vi "user32_GetMessage.vi"(5 "wMsgFilterMax":u32, 7 "wMsgFilterMin":u32, 8 "错误输入（无错误）":errorcluster, 10 "lpMsg":u32, 11 "hWnd":u32) -> (0 "错误输出":errorcluster, 2 "success?":bool, 3 "dup hWnd":u32)   [LabVIEW 2011]
doc: "函数GetMessage是从调用线程的消息队列里取得一个消息并将其放于指定的结构。此函数可取得与指定窗口联系的消息和由PostThreadMesssge寄送的线程消息。此函数接收一定范围的消息值。GetMessage不接收属于其他线程或应用程序的消息。获取消息成功后，线程将从消息队列中删除该消息。函数会一直等待直到有消息到来才有返回值。"
uses:
  user32.dll
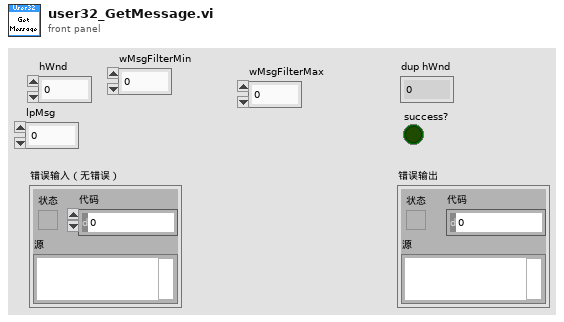
[diagram p1: front panel]
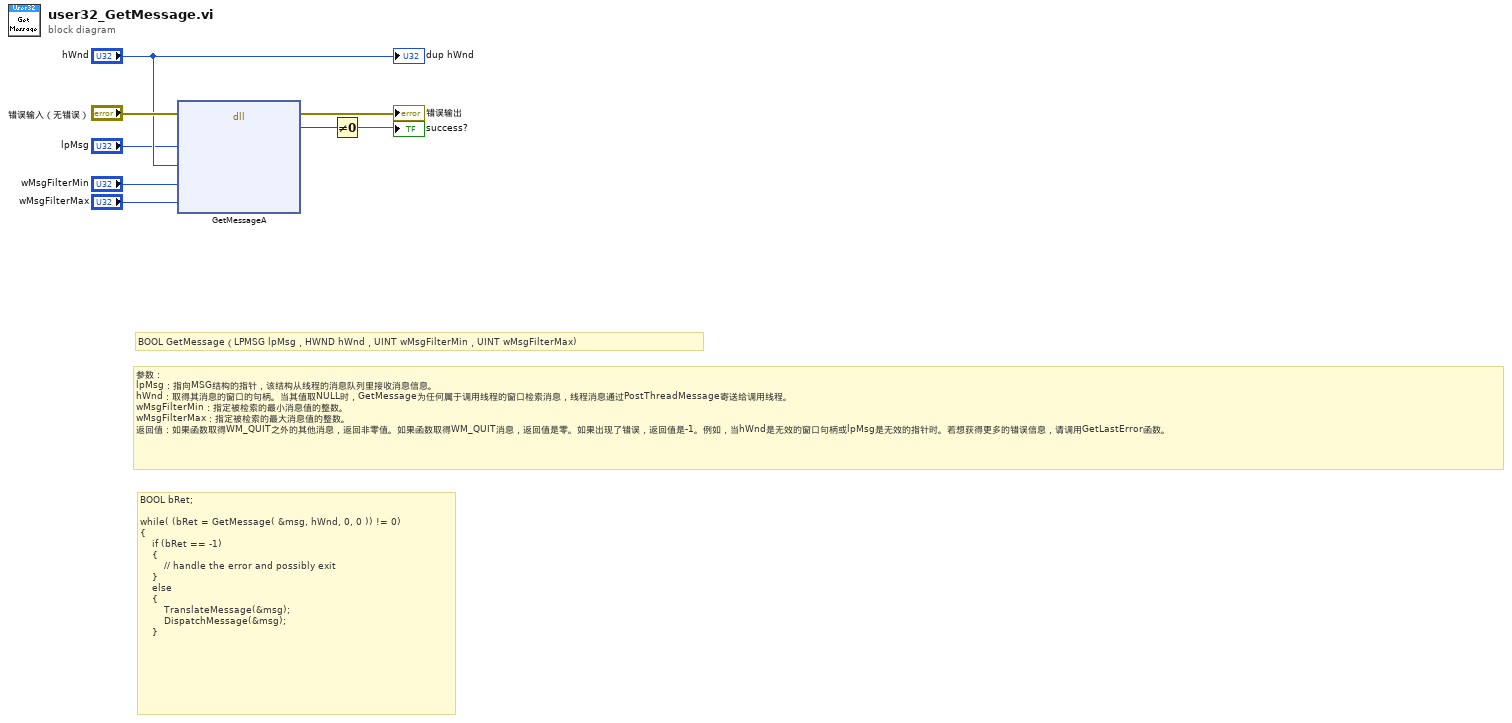
[diagram p0: block diagram]
diagram:
  # "BOOL bRet;\n \nwhile( (bRet = GetMessage( &msg, hWnd, 0, 0 )) != 0)\n{ \n    if (bRet == -1)\n    {\n        // handle the error and possibly exit\n    }\n    else\n    {\n        TranslateMessage(&msg); \n        DispatchMessage(&msg); \n    }"
  # "参数：\nlpMsg：指向MSG结构的指针，该结构从线程的消息队列里接收消息信息。\nhWnd：取得其消息的窗口的句柄。当其值取NULL时，GetMessage为任何属于调用线程的窗口检索消息，线程消息通过PostThreadMessage寄送给调用线程。\nwMsgFilterMin：指定被检索的最小消息值的整数。\nwMsgFilterMax：指定被检索的最大消息值的整数。\n返回值：如果函数取得WM_QUIT之外的其他消息，返回非零值。如果函数取得WM_QUIT消息，返回值是零。如果出现了错误，返回值是-1。例如，当hWnd是无效的窗口句柄或lpMsg是无效的指针时。若想获得更多的错误信息，请调用GetLastError函数。"
  # "BOOL GetMessage（LPMSG lpMsg，HWND hWnd，UINT wMsgFilterMin，UINT wMsgFilterMax)"
  n1 = dll-call lib="user32.dll" fn="GetMessageA"(error in="错误输入（无错误）", "lpMsg"="lpMsg", "hWnd"="hWnd", "wMsgFilterMin"="wMsgFilterMin", "wMsgFilterMax"="wMsgFilterMax") -> (error out=→"错误输出":errorcluster, "Bool"=w5:i32)  [unwired: 6 in, 1 out]
  n2 = Not Equal To 0?(x=w5) -> (x != 0?=→"success?":bool)
  "dup hWnd" <- "hWnd"
